vi "read_counter.vi"() -> ()   [LabVIEW 2013]
uses:
  <vilib>/DAQmx/read.llb/DAQmx Read.vi
  <vilib>/DAQmx/read.llb/DAQmx Read (Counter DBL 1Chan 1Samp).vi
  <vilib>/DAQmx/miscellaneous.llb/DAQmx Fill In Error Info.vi
panel:
  in  "stop":bool caption="停止"
  out "data":dbl caption="数据" format="%#_6p"
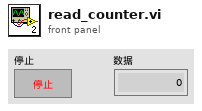
[diagram p1: front panel]
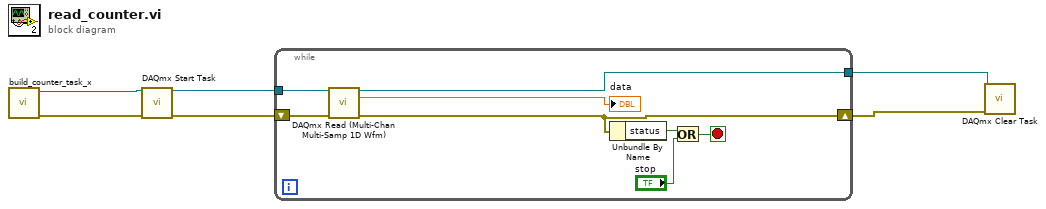
[diagram p0: block diagram]
diagram:
  n1 = call "build_counter_task_x.vi"() -> ("error out"=w1:errorcluster, "task out"=w2:refnum<k21>)  [unwired: 10 in]
  n2 = call <vilib>:"DAQmx Start Task.vi"("task/channels in"=w2, "error in"=w1) -> ("task out"=w6:refnum<k21>, "error out"=w5:errorcluster)  [unwired: 12 in]
  n3 = while "While循环" {
    tunnel: w6 -> [w14]
    tunnel: [w12] -> w3
    shift-right: [w7] -> w4
    shift-left: w5 -> [w13]
    stop <- w8 stop-if-true
    n4 = call-poly "DAQmx Read (Multi-Chan Multi-Samp 1D Wfm).vi"("task/channels in"=w14, "error in"=w13) -> ("task out"=w12:refnum<k21>, "data"=→"data":dbl, "error out"=w7:errorcluster)  [unwired: 11 in]
    n5 = Unbundle By Name(w7) -> ("status"=w10:bool)
    n6 = Or(x=w10, y="stop") -> (x .or. y?=w8:bool)
  }
  n7 = call <vilib>:"DAQmx Clear Task.vi"("task in"=w3, "error in"=w4) -> ()  [unwired: 13 in, 1 out]
